vi "Jeffress_model_v007.vi"() -> ()   [LabVIEW 2019]
panel:
  out "Elapsed time 2":dbl caption="Get Start Time (s)"
  out "new picture":picture
  out "Left - Right":dbl
  out "Elapsed time 1":dbl caption="Get Start Time (s)"
  in  "stop":bool
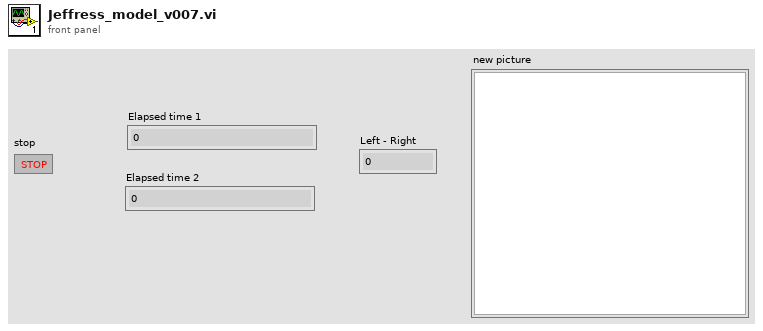
[diagram p1: front panel]
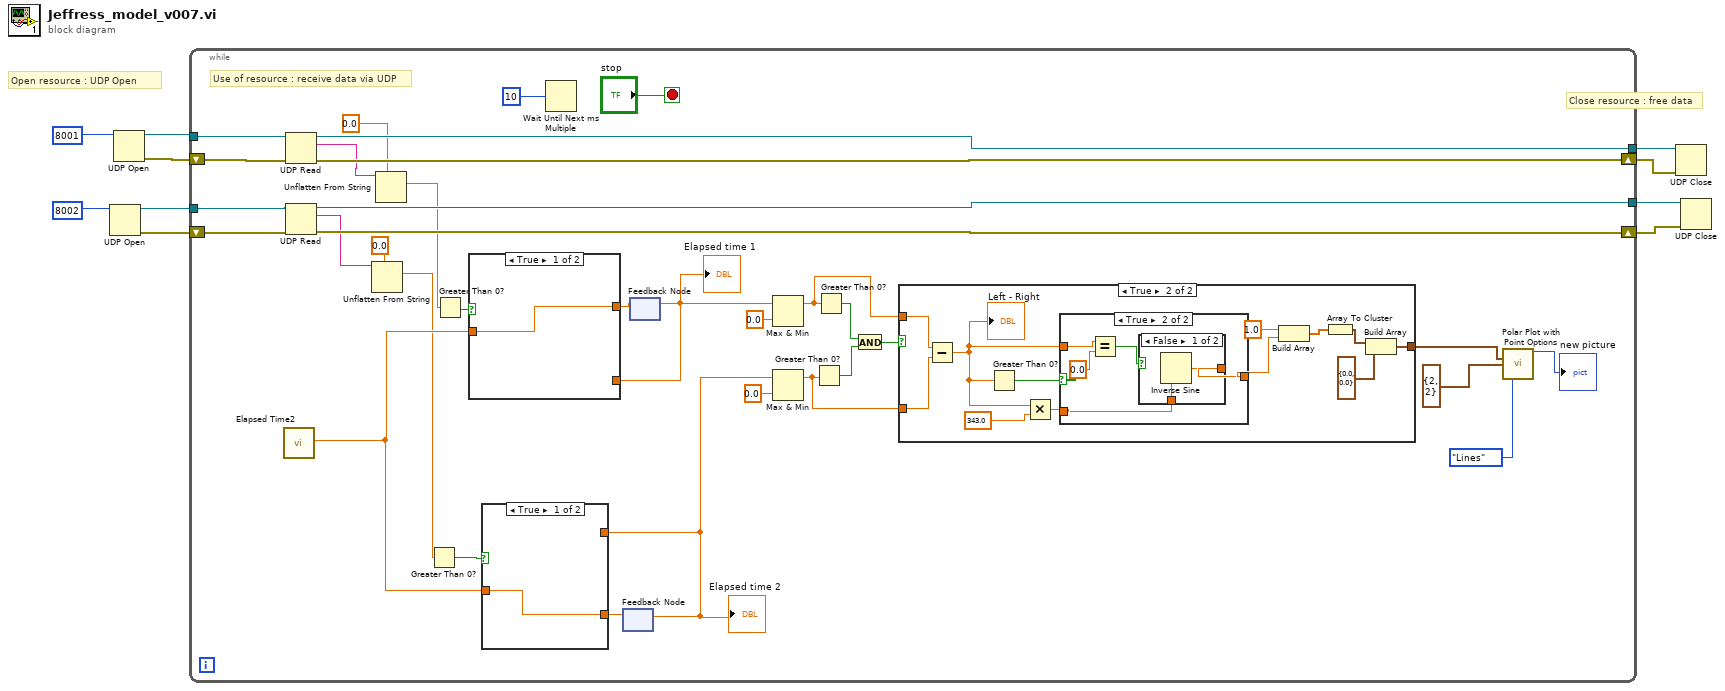
[diagram p0: block diagram]
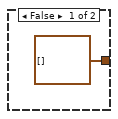
[diagram p3: hidden frame]
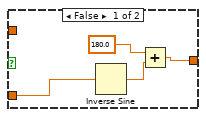
[diagram p4: hidden frame]
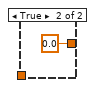
[diagram p5: hidden frame]
diagram:
  # "Close resource : free data"
  # "Open resource : UDP Open"
  n1 = UDP Open(11:u16 8002) -> (port=w4:refnum<k16>, 0:w1:errorcluster)  [unwired: 4 in, 1 out]
  n2 = UDP Open(11:u16 8001) -> (port=w8:refnum<k16>, 0:w10:errorcluster)  [unwired: 4 in, 1 out]
  n3 = while {
    tunnel: w8 -> [w40]
    tunnel: [w39] -> w7
    shift-right: [w42] -> w9
    shift-left: w10 -> [w41]
    tunnel: w4 -> [w28]
    tunnel: [w26] -> w2
    shift-right: [w27] -> w3
    shift-left: w1 -> [w25]
    stop <- "stop" stop-if-true
    # "Use of resource : receive data via UDP"
    n4 = call "Elapsed Time2"() -> ("Elapsed Time (s)"=w23:dbl)  [unwired: 12 in, 7 out]
    n5 = UDP Read(connection ID=w40, 8:w41) -> (data out=w18:string, error out=w42:errorcluster, 3:w39:refnum<k16>)  [unwired: 2 in, 2 out]
    n6 = UDP Read(connection ID=w28, 8:w25) -> (data out=w13:string, error out=w27:errorcluster, 3:w26:refnum<k16>)  [unwired: 2 in, 2 out]
    n7 = Unflatten From String(type=0.0 ("y"), binary string=w13) -> (value=w11:dbl)  [unwired: 3 in, 2 out]
    n8 = Unflatten From String(type=0.0 ("y"), binary string=w18) -> (value=w15:dbl)  [unwired: 3 in, 2 out]
    n9 = Greater Than 0?(x=w11) -> (x > 0?=w12:bool)
    n10 = Greater Than 0?(x=w15) -> (x > 0?=w17:bool)
    n11 = Wait Until Next ms Multiple(millisecond multiple=u32 10) -> ()  [unwired: 1 out]
    n12 = feedback #1() -> (w19:dbl)  [unwired: 1 in]
    "Elapsed time 2" <- w19
    n13 = case shown="True" w12 {
      tunnel: w23 -> [w72 _]
      tunnel: [w72 w73] -> w22
      tunnel: w19 -> [_ w73]
      frame True {
      }
      frame False {
      }
    }
    n14 = feedback-in #1(w22) -> ()
    n15 = feedback #2() -> (w20:dbl)  [unwired: 1 in]
    "Elapsed time 1" <- w20
    n16 = case shown="True" w17 {
      tunnel: w23 -> [w45 _]
      tunnel: [w45 w46] -> w21
      tunnel: w20 -> [_ w46]
      frame True {
      }
      frame False {
      }
    }
    n17 = feedback-in #2(w21) -> ()
    n18 = Max & Min(x=w20, y=0.0) -> (max(x,y)=w33:dbl)  [unwired: 1 out]
    n19 = Max & Min(x=w19, y=0.0) -> (max(x,y)=w34:dbl)  [unwired: 1 out]
    n20 = Greater Than 0?(x=w34) -> (x > 0?=w35:bool)
    n21 = Greater Than 0?(x=w33) -> (x > 0?=w36:bool)
    n22 = And(x=w36, y=w35) -> (x .and. y?=w24:bool)
    n23 = case shown="True" w24 {
      tunnel: w33 -> [_ w58]
      tunnel: w34 -> [_ w59]
      tunnel: [cluster{"[0]":dbl, "[1]":dbl}[] [] w53] -> w32
      frame False {
      }
      frame True {
        n24 = Subtract(x=w58, y=w59) -> (x-y=w48:dbl)
        "Left - Right" <- w48
        n25 = Greater Than 0?(x=w48) -> (x > 0?=w57:bool)
        n26 = Multiply(x=w48, y=343.0) -> (x*y=w52:dbl)
        n27 = case shown="True" w57 {
          tunnel: w52 -> [w63 w67]
          tunnel: [w62 w68] -> w51
          tunnel: w48 -> [_ w64]
          frame False {
            n28 = Inverse Sine(1:w63) -> (0:w61:dbl)
            n29 = Add(x=180.0, y=w61) -> (x+y=w62:dbl)
          }
          frame True {
            n30 = Equal?(x=w64, y=0.0 ("x")) -> (x = y?=w66:bool)
            n31 = case shown="False" w66 {
              tunnel: [w70 0.0] -> w68
              tunnel: w67 -> [w69 _]
              frame False {
                n32 = Inverse Sine(1:w69) -> (0:w70:dbl)
              }
              frame True {
              }
            }
          }
        }
        n33 = Build Array(1.0 ("element"), w51) -> (w55:dbl[])
        n34 = Array To Cluster(array=w55) -> (cluster=w54:cluster{"[0]":dbl, "[1]":dbl})
        n35 = Build Array(w54, cluster{"[0]":dbl, "[1]":dbl} {"[0]"=0.0, "[1]"=0.0} ("element")) -> (w53:cluster{"[0]":dbl, "[1]":dbl}[])
      }
    }
    n36 = call <vilib>:"Polar Plot with Point Options.vi"("data array [mag, phase (deg)]"=w32, "top left point(0, 0)"=cluster{"x":i16, "y":i16} {"x"=2, "y"=2}, "Lines/Points"=enum16{"Lines", "Points"}."Lines") -> ("new picture"=→"new picture":picture)  [unwired: 12 in]
  }
  n37 = UDP Close(connection ID=w7, 8:w9) -> ()  [unwired: 2 out]
  n38 = UDP Close(connection ID=w2, 8:w3) -> ()  [unwired: 2 out]
